vi "TDMS File Writer And Close.vi"(11 "TDMS Cluster":T1) -> ()   [LabVIEW 2015]
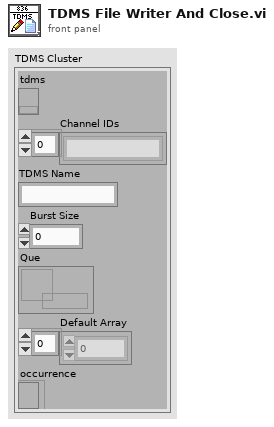
[diagram p1: front panel]
types:
  T1 = cluster{"tdms":refnum<k34>, "Channel IDs":string[], "TDMS Name":string, "Burst Size":i32, "Que":refnum<k33>, "Default Array":dbl[], "occurrence":refnum<k4>}
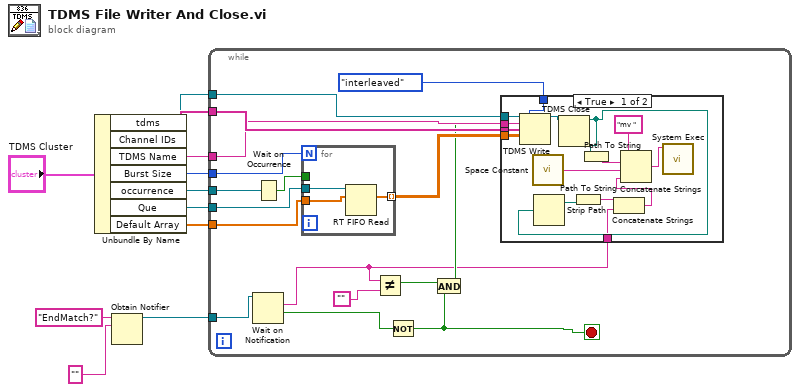
[diagram p0: block diagram]
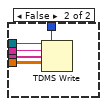
[diagram p2: hidden frame]
diagram:
  n1 = Unbundle By Name("TDMS Cluster") -> ("tdms"=w4:refnum<k34>, "Channel IDs"=w5:string[], "TDMS Name"=w6:string, "Burst Size"=w7:i32, "occurrence"=w8:refnum<k4>, "Que"=w9:refnum<k33>, "Default Array"=w10:dbl[])
  n2 = Obtain Notifier(name (unnamed)="EndMatch?", notification data type="") -> (notifier out=w3:refnum<notifier>)  [unwired: 2 in, 2 out]
  n3 = while {
    tunnel: w8 -> [w22]
    tunnel: w9 -> [w28]
    tunnel: w10 -> [w27]
    tunnel: w5 -> [w26]
    tunnel: w6 -> [w25]
    tunnel: w4 -> [w24]
    tunnel: w7 -> [w23]
    tunnel: w3 -> [w18]
    stop <- w12 stop-if-true
    n4 = Wait on Notification(notifier=w18) -> (notification=w15:string, timed out?=w13:bool)  [unwired: 3 in, 2 out]
    n5 = Wait on Occurrence(2:w22) -> (0:w19:bool)  [unwired: 2 in]
    n6 = for {
      N: w23 -> [_]
      tunnel: w28 -> [w51]
      tunnel: w27 -> [w50]
      tunnel: [w49] -> w21 mode=indexing
      tunnel: w19 -> [_]
      n7 = RT FIFO Read(0:w51, 1:w50) -> (9:w49:dbl[])  [unwired: 2 in, 4 out]
    }
    n8 = Not Equal?(x=w15, y="") -> (x != y?=w16:bool)
    n9 = Not(x=w13) -> (.not. x?=w12:bool)
    n10 = And(x=w16, y=w12) -> (x .and. y?=w17:bool)
    n11 = case shown="True" w17 {
      tunnel: w26 -> [w43 w48]
      tunnel: w25 -> [w42 w47]
      tunnel: w24 -> [w41 w46]
      tunnel: w21 -> [w40 w45]
      tunnel: enum16{"decimated", "interleaved"}."interleaved" ("data layout (0:decimated)") -> [w39 w44]
      tunnel: w15 -> [w31 _]
      frame True {
        n12 = TDMS Write(0:w41, 1:w39, 5:w42, 7:w43, 9:w40) -> (4:w38:refnum<k34>)  [unwired: 1 in, 3 out]
        n13 = call <vilib>:"Space Constant.vi"() -> ("String"=w29:string)
        n14 = TDMS Close(11:w38) -> (3:w34:path)  [unwired: 1 in, 1 out]
        n15 = Strip Path(path=w34) -> (stripped path=w33:path)  [unwired: 1 out]
        n16 = Path To String(path=w33) -> (string=w32:string)
        n17 = Path To String(path=w34) -> (string=w35:string)
        n18 = Concatenate Strings(w32, w31) -> (w30:string)
        n19 = Concatenate Strings("mv ", w35, w29, w30) -> (w37:string)
        n20 = call <vilib>:"System Exec.vi"("command line"=w37) -> ()  [unwired: 7 in, 4 out]
      }
      frame False {
        n21 = TDMS Write(0:w46, 1:w44, 5:w47, 7:w48, 9:w45) -> ()  [unwired: 1 in, 4 out]
      }
    }
  }
